vi "AlliGator Draw Tick Labels.vi"(4 "Label Distance (tick unit)":dbl=2.0, 5 "Font, Size & Style":T4, 6 "Text Color":u32, 7 "Overlay Group":string, 8 "error in (no error)":errorcluster, 9 "Phasor Plot Reference Points":T5, 10 "Tick Label Data":T1[](array[typedef]), 11 "Refnum in":T3) -> (0 "error out":errorcluster, 3 "Refnum out":T3)   [LabVIEW 2021, in "AlliGator Phasor Plot.lvlib"]
doc: "Draws UC or SEPL tick labels in the Phasor Plot image."
uses:
  AlliGator Phasor Plot.lvlib
  AlliGator Phasor Plot Reference Points.ctl
  <vilib>/vision/Image Controls.llb/IMAQ Image.ctl
  Phasor/Phasor SEPL Tick Data.ctl
  Phasor/Phasor (g, s).ctl
  Strings/Strings.lvlib
  AlliGator Phasor Ratio.lvlib
  Phasor/Phasor.lvlib
panel:
  # "see the AlliGator License on the block diagram (Ctrl+E or Window:Show Block Diagram)"
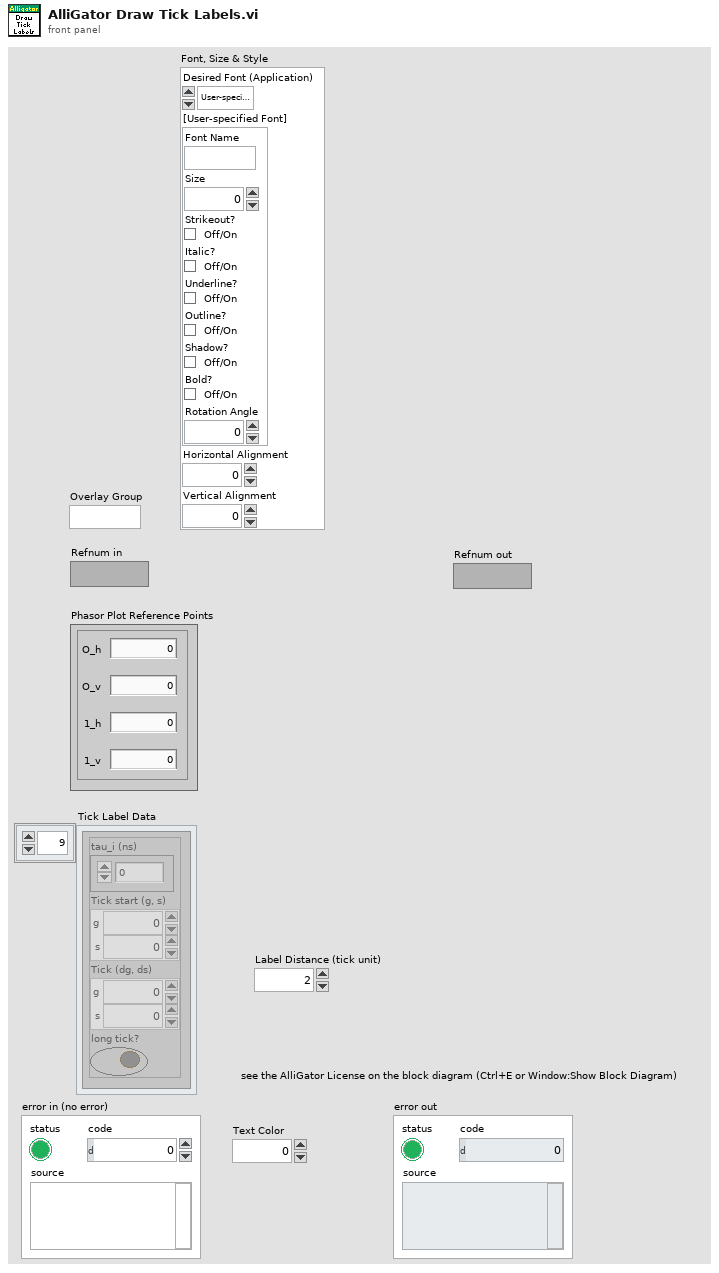
[diagram p1: front panel]
types:
  T1 = typedef "Phasor.lvlib/Phasor SEPL Tick Data.ctl" = cluster{"tau_i (ns)":dbl, "Tick start (g, s)":T2, "Tick (dg, ds)":T2, "long tick?":bool}
  T2 = typedef "Phasor.lvlib/Phasor (g, s).ctl" = cluster{"g":dbl, "s":dbl}
  T3 = typedef "IMAQ Image.ctl" = refnum<image>
  T4 = cluster{"Desired Font (Application)":enum16{"User-specified Font", "Application Font", "System Font", "Dialog Font"}, "[User-specified Font]":cluster{"Font Name":string, "Size":i16, "Strikeout?":bool, "Italic?":bool, "Underline?":bool, "Outline?":bool, "Shadow?":bool, "Bold?":bool, "Rotation Angle":dbl}, "Horizontal Alignment":i16, "Vertical Alignment":i16}
  T5 = typedef "AlliGator Phasor Ratio.lvlib/AlliGator Phasor Plot Reference Points.ctl" = cluster{"O_h":dbl, "O_v":dbl, "1_h":dbl, "1_v":dbl}
  T6 = cluster{"Phasor Plot x":dbl, "Phasor Plot y":dbl}
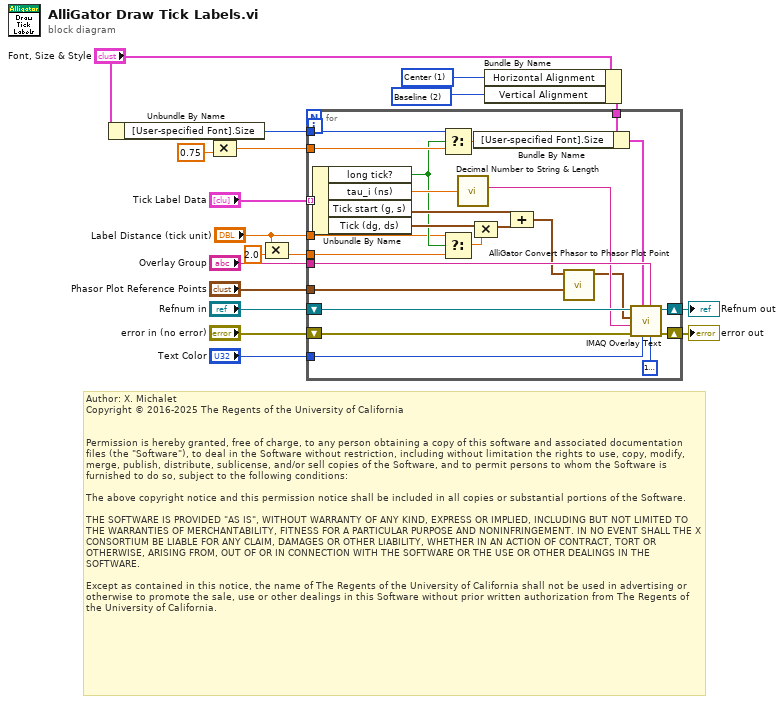
[diagram p0: block diagram]
diagram:
  w8 = i16 2 items=["Bottom", "Top", "Baseline"] ("Vertical Alignment")
  w9 = i16 1 items=["Left", "Center", "Right"] ("Horizontal Alignment")
  # "Author: X. Michalet\nCopyright © 2016-2025 The Regents of the University of California\n \n\nPermission is hereby granted, free of charge, to any person obtaining a copy of this software and associated documentation files (the \"Software\"), to deal in the Software without restriction, including without limitation the rights to use, copy, modify, merge, publish, distribute, sublicense, and/or sell copies of the Software, and to permit persons to whom the Software is furnished to do so, subject to the following conditions:\n\nThe above copyright notice and this permission notice shall be included in all copies or substantial portions of the Software.\n\nTHE SOFTWARE IS PROVIDED \"AS IS\", WITHOUT WARRANTY OF ANY KIND, EXPRESS OR IMPLIED, INCLUDING BUT NOT LIMITED TO THE WARRANTIES OF MERCHANTABILITY, FITNESS FOR A PARTICULAR PURPOSE AND NONINFRINGEMENT. IN NO EVENT SHALL THE X CONSORTIUM BE LIABLE FOR ANY CLAIM, DAMAGES OR OTHER LIABILITY, WHETHER IN AN ACTION OF CONTRACT, TORT OR OTHERWISE, ARISING FROM, OUT OF OR IN CONNECTION WITH THE SOFTWARE OR THE USE OR OTHER DEALINGS IN THE SOFTWARE.\n\nExcept as contained in this notice, the name of The Regents of the University of California shall not be used in advertising or otherwise to promote the sale, use or other dealings in this Software without prior written authorization from The Regents of the University of California."
  n1 = Unbundle By Name("Font, Size & Style") -> ("[User-specified Font].Size"=w6:i16)
  n2 = Compound Arithmetic op=MULTIPLY(w6, 0.75 ("value")) -> (w4:dbl)
  n3 = Compound Arithmetic op=MULTIPLY("Label Distance (tick unit)", 2.0 ("s? t:f")) -> (w2:dbl)
  n4 = Bundle By Name(cluster="Font, Size & Style", "Horizontal Alignment"=w9, "Vertical Alignment"=w8) -> (w10:T4)
  n5 = for {
    shift-right: [w38] -> w13
    shift-left: "Refnum in" -> [w39]
    shift-right: [w42] -> w15
    shift-left: "error in (no error)" -> [w43]
    tunnel: "Tick Label Data" -> [w36] mode=indexing
    tunnel: "Text Color" -> [w41]
    tunnel: "Overlay Group" -> [w40]
    tunnel: w10 -> [w37]
    tunnel: "Phasor Plot Reference Points" -> [w32]
    tunnel: w6 -> [w24]
    tunnel: w4 -> [w23]
    tunnel: "Label Distance (tick unit)" -> [w20]
    tunnel: w2 -> [w19]
    n6 = Unbundle By Name(w36) -> ("long tick?"=w21:bool, "tau_i (ns)"=w29:dbl, "Tick start (g, s)"=w35:T2, "Tick (dg, ds)"=w34:T2)
    n7 = Select(t=w24, s=w21, f=w23) -> (s? t:f=w25:dbl)
    n8 = Select(t=w20, s=w21, f=w19) -> (s? t:f=w22:dbl)
    n9 = call "Decimal Number to String & Length.vi"("Decimal Number"=w29) -> ("String"=w28:string)  [unwired: 6 in, 1 out]
    n10 = Bundle By Name(cluster=w37, "[User-specified Font].Size"=w25) -> (w26:T4)
    n11 = Compound Arithmetic op=MULTIPLY(w34, w22) -> (w33:T2)
    n12 = Compound Arithmetic op=ADD(w35, w33) -> (w31:T2)
    n13 = call "AlliGator Convert Phasor to Phasor Plot Point.vi"("Phasor Plot Reference Points"=w32, "Phasor"=w31) -> ("Phasor Plot Point"=w27:T6)  [unwired: 9 in]
    n14 = call "IMAQ Overlay Text"("BG Color (Transparent)"=u32 16777216, "Group"=w40, "Text Color (black)"=w41, "Font, Size & Style"=w26, "error in (no error)"=w43, "String"=w28, "Origin"=w27, "Image"=w39) -> ("error out"=w42:errorcluster, "Image Out"=w38:T3)  [unwired: 2 in]
  }
  "error out" <- w15
  "Refnum out" <- w13
